vi "shell integration.vi"(7 "Command":enum16{"Add", "Remove"}(ring)=enum."Remove", 8 "error in":errorcluster, 11 "Cluster":T1={"App Key"="Test Key", "Context Label"="Test File Roottt", "Command"="Cmd", "Position"=enum."Middle", "Extended?"=FALSE, "Location"=enum."File - Root", "Icon path"="\"C:\\Users\\sajam\\LabVIEW Projects\\Personal projects\\Rename Extension\\Source Code\\rename.ico\"", "Ext (No Dot)"="Test"}) -> (0 "error out":errorcluster, 3 "Cluster":T1={"App Key"="Test Key", "Context Label"="Test Command", "Command"="none", "Position"=enum."Middle", "Extended?"=FALSE, "Location"=enum."Ext - Classes", "Icon path"="\"C:\\Users\\sajam\\LabVIEW Projects\\Personal projects\\Rename Extension\\Source Code\\rename.ico\"", "Ext (No Dot)"="Test"})   [LabVIEW 2023, in "User Interface.lvlib"]
uses:
  User Interface.lvlib
  Controls/registry settings cluster.ctl
  <vilib>/registry/registry.llb/Registry RtKey.ctl
  <vilib>/registry/registry.llb/Write Registry Value Simple STR.vi
panel:
  out "standard error":string
  out "standard output":string
  out "String":string
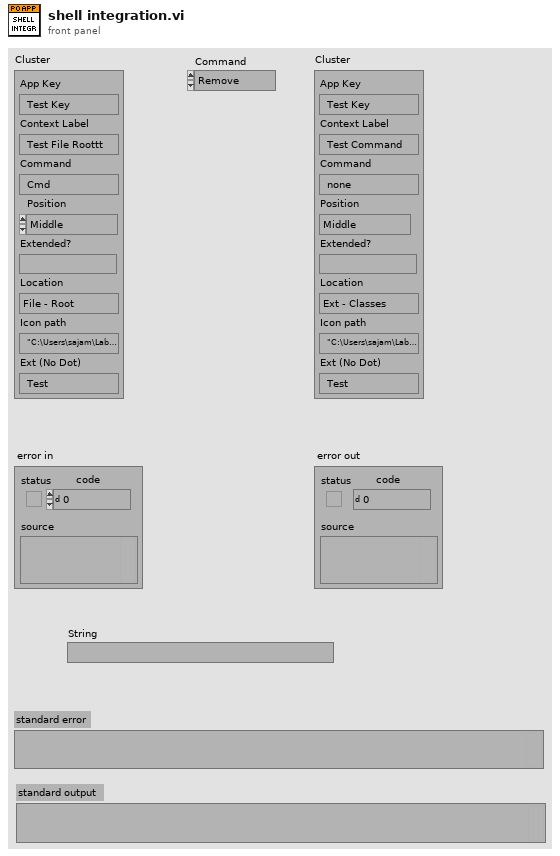
[diagram p1: front panel]
types:
  T1 = typedef "User Interface.lvlib/registry settings cluster.ctl" = cluster{"App Key":string, "Context Label":string, "Command":string, "Position":enum16{"Top", "Middle", "Bottom"}, "Extended?":bool, "Location":enum16{"File - Root", "Ext - Root", "Directory - Root", "File - Classes", "Ext - Classes", "Folder - Classes", "Dir Bak Gnd - Root"}, "Icon path":string, "Ext (No Dot)":string}
  T2 = typedef "Registry RtKey.ctl" = enum32{"HKEY_CLASSES_ROOT", "HKEY_CURRENT_USER", "HKEY_LOCAL_MACHINE", "HKEY_USERS", "HKEY_PERFORMANCE_DATA", "HKEY_CURRENT_CONFIG", "HKEY_DYN_DATA"}
  T3 = enum16{"File - Root", "Ext - Root", "Directory - Root", "File - Classes", "Ext - Classes", "Folder - Classes", "Dir Bak Gnd - Root"}
  T4 = typedef "Registry refnum.ctl" = refnum<k1>
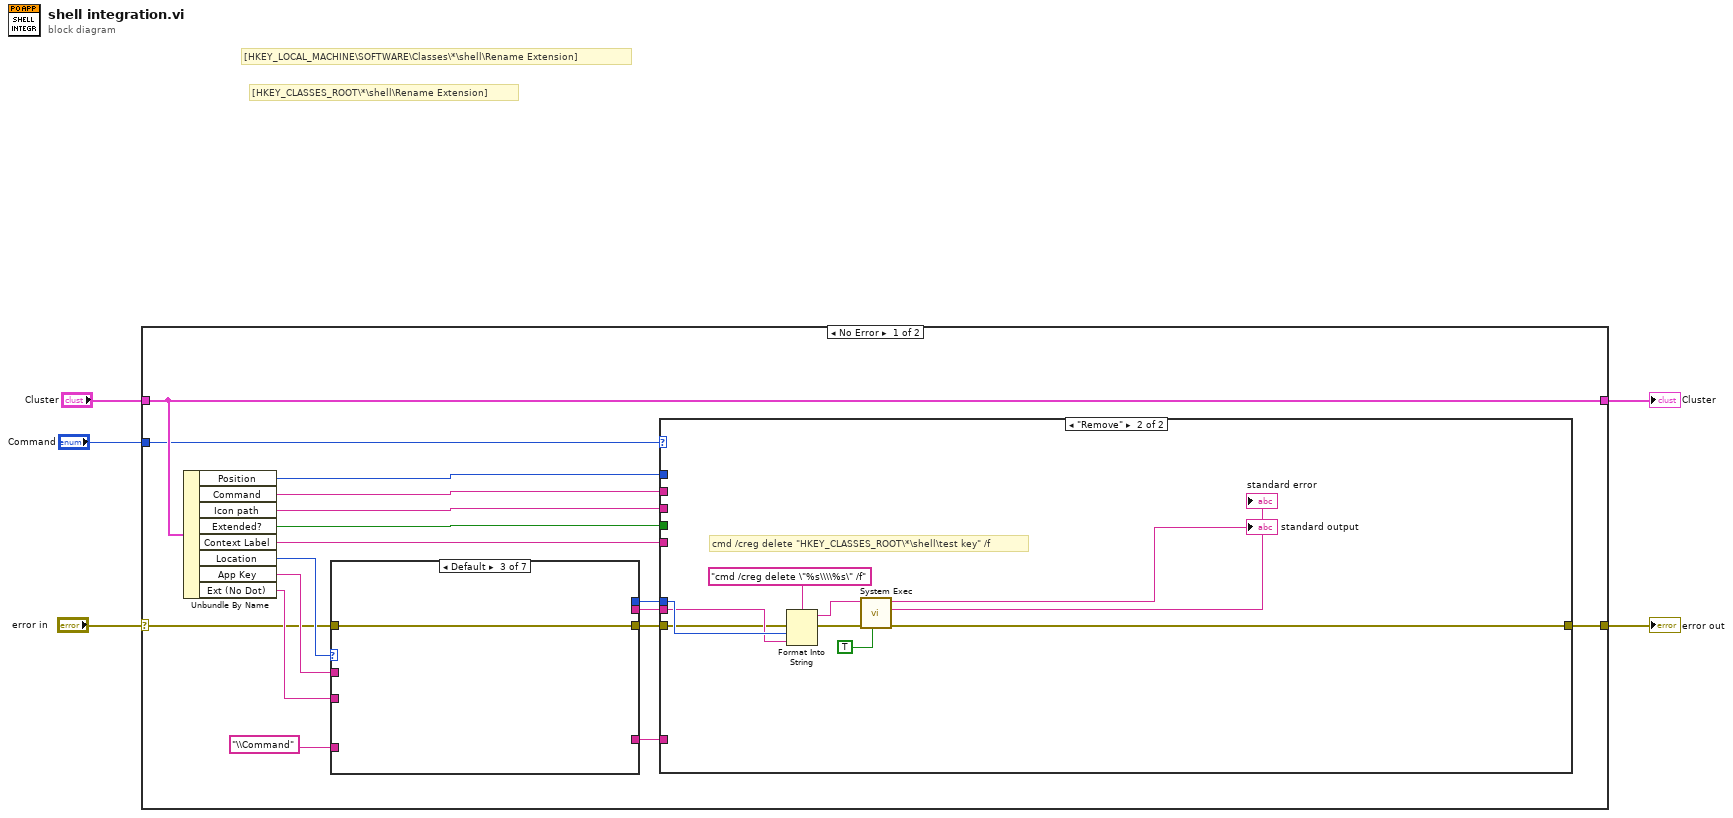
[diagram p0: block diagram]
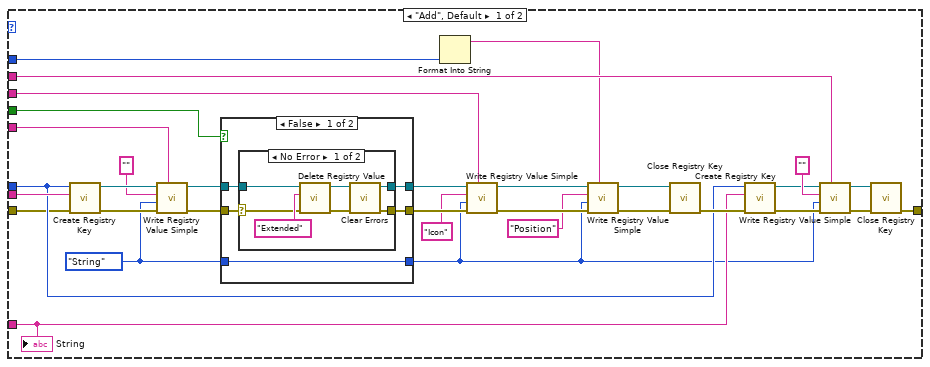
[diagram p2: hidden frame]
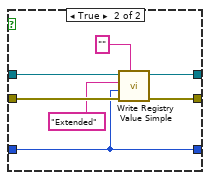
[diagram p4: hidden frame]
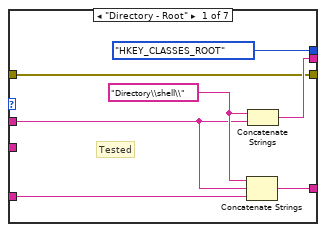
[diagram p5: hidden frame]
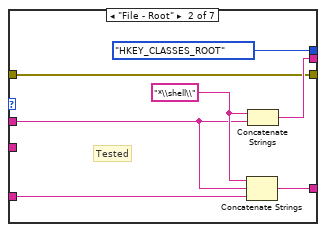
[diagram p6: hidden frame]
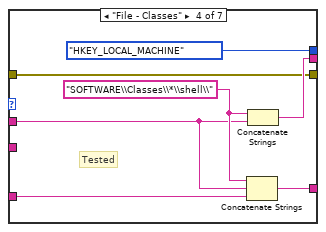
[diagram p7: hidden frame]
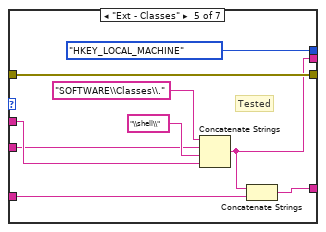
[diagram p8: hidden frame]
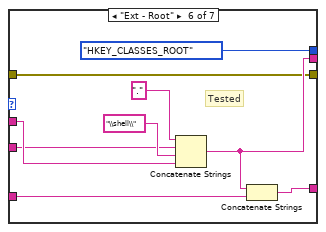
[diagram p9: hidden frame]
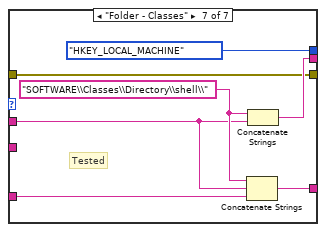
[diagram p10: hidden frame]
diagram:
  # "[HKEY_CLASSES_ROOT\\*\\shell\\Rename Extension]"
  # "[HKEY_LOCAL_MACHINE\\SOFTWARE\\Classes\\*\\shell\\Rename Extension]"
  n1 = case shown="No Error" "error in" {
    selector: "error in" -> [w9 w133]
    tunnel: "Cluster" -> [w8 w132]
    tunnel: [w6 w133] -> w4
    tunnel: [w8 w132] -> w2
    tunnel: "Command" -> [w7 _]
    frame No Error {
      n2 = Unbundle By Name(w8) -> ("Position"=w10:enum16{"Top", "Middle", "Bottom"}, "Command"=w15:string, "Icon path"=w14:string, "Extended?"=w18:bool, "Context Label"=w19:string, "Location"=w21:T3, "App Key"=w20:string, "Ext (No Dot)"=w12:string)
      n3 = case shown="Default" w21 {
        tunnel: [Registry_RtKey."HKEY_CLASSES_ROOT" ("root key (HKEY_LOCAL_MACHINE)") Registry_RtKey."HKEY_CLASSES_ROOT" ("root key (HKEY_LOCAL_MACHINE)") _ Registry_RtKey."HKEY_LOCAL_MACHINE" ("root key (HKEY_LOCAL_MACHINE)") Registry_RtKey."HKEY_LOCAL_MACHINE" ("root key (HKEY_LOCAL_MACHINE)") Registry_RtKey."HKEY_CLASSES_ROOT" ("root key (HKEY_LOCAL_MACHINE)") Registry_RtKey."HKEY_LOCAL_MACHINE" ("root key (HKEY_LOCAL_MACHINE)")] -> w17
        tunnel: [w90 w97 _ w105 w107 w117 w130] -> w22
        tunnel: w20 -> [w88 w95 _ w103 w113 w122 w128]
        tunnel: [w87 w94 _ w102 w112 w121 w127] -> w16
        tunnel: "\\Command" ("string") -> [w86 w93 _ w101 w111 w120 w126]
        tunnel: w12 -> [_ _ _ _ w110 w118 _]
        tunnel: w9 -> [w85 w92 w99 w100 w108 w116 w125]
        tunnel: [w85 w92 w99 w100 w108 w116 w125] -> w11
        frame "Directory - Root" {
          w89 = "Directory\\shell\\" ("subkey")
          # "Tested"
          n4 = Concatenate Strings(w89, w88, w86) -> (w87:string)
          n5 = Concatenate Strings(w89, w88) -> (w90:string)
        }
        frame "File - Root" {
          w96 = "*\\shell\\" ("subkey")
          # "Tested"
          n6 = Concatenate Strings(w96, w95, w93) -> (w94:string)
          n7 = Concatenate Strings(w96, w95) -> (w97:string)
        }
        frame Default {
        }
        frame "File - Classes" {
          w104 = "SOFTWARE\\Classes\\*\\shell\\" ("subkey")
          # "Tested"
          n8 = Concatenate Strings(w104, w103, w101) -> (w102:string)
          n9 = Concatenate Strings(w104, w103) -> (w105:string)
        }
        frame "Ext - Classes" {
          # "Tested"
          n10 = Concatenate Strings("SOFTWARE\\Classes\\." ("subkey"), w110, "\\shell\\" ("subkey"), w113) -> (w107:string)
          n11 = Concatenate Strings(w107, w111) -> (w112:string)
        }
        frame "Ext - Root" {
          # "Tested"
          n12 = Concatenate Strings("." ("subkey"), w118, "\\shell\\" ("subkey"), w122) -> (w117:string)
          n13 = Concatenate Strings(w117, w120) -> (w121:string)
        }
        frame "Folder - Classes" {
          w129 = "SOFTWARE\\Classes\\Directory\\shell\\" ("subkey")
          # "Tested"
          n14 = Concatenate Strings(w129, w128, w126) -> (w127:string)
          n15 = Concatenate Strings(w129, w128) -> (w130:string)
        }
      }
      n16 = case shown="\"Remove\"" w7 {
        tunnel: w22 -> [w54 w80]
        tunnel: w19 -> [w51 _]
        tunnel: w18 -> [w48 _]
        tunnel: w17 -> [w39 w81]
        tunnel: w16 -> [w38 _]
        tunnel: w15 -> [w36 _]
        tunnel: [w23 w77] -> w6
        tunnel: w14 -> [w35 _]
        tunnel: w11 -> [w34 w79]
        tunnel: w10 -> [w29 _]
        frame "Add", Default {
          w47 = enum16{"String", "Binary", "DWORD"}."String" ("simple data type")
          n17 = call <vilib>:"Create Registry Key.vi"("error in (no error)"=w34, "subkey"=w54, "root key (HKEY_LOCAL_MACHINE)"=w39) -> ("error out"=w52:errorcluster, "refnum out"=w53:T4)  [unwired: 6 in, 1 out]
          n18 = call-poly <vilib>:"Write Registry Value Simple.vi"("String/Binary data"=w51, "error in (no error)"=w52, "simple data type"=w47, "value"="", "refnum"=w53) -> ("error out"=w49:errorcluster, "refnum out"=w50:T4)  [unwired: 3 in]
          n19 = case shown="False" w48 {
            tunnel: w50 -> [w57 w74]
            tunnel: w49 -> [w58 w73]
            tunnel: [w56 w71] -> w45
            tunnel: [w55 w70] -> w46
            tunnel: w47 -> [w59 w69]
            tunnel: [w59 w69] -> w26
            frame False {
              n20 = case shown="No Error" w58 {
                selector: w58 -> [w60 w67]
                tunnel: w57 -> [w64 w66]
                tunnel: [w63 w66] -> w56
                tunnel: [w61 w67] -> w55
                frame No Error {
                  n21 = call <vilib>:"Delete Registry Value.vi"("error in (no error)"=w60, "value"="Extended", "refnum"=w64) -> ("error out"=w65:errorcluster, "refnum out"=w63:T4)  [unwired: 7 in]
                  n22 = call <vilib>:"Clear Errors.vi"("error in (no error)"=w65) -> ("error out"=w61:errorcluster)  [unwired: 5 in, 1 out]
                }
                frame Error {
                }
              }
            }
            frame True {
              n23 = call-poly <vilib>:"Write Registry Value Simple.vi"("String/Binary data"="", "error in (no error)"=w73, "simple data type"=w69, "value"="Extended", "refnum"=w74) -> ("error out"=w70:errorcluster, "refnum out"=w71:T4)  [unwired: 3 in]
            }
          }
          n24 = Format Into String(w29) -> (resulting string=w28:string)  [unwired: 3 in, 1 out]
          n25 = call-poly <vilib>:"Write Registry Value Simple.vi"("String/Binary data"=w35, "error in (no error)"=w46, "simple data type"=w26, "value"="Icon", "refnum"=w45) -> ("error out"=w33:errorcluster, "refnum out"=w31:T4)  [unwired: 3 in]
          n26 = call-poly <vilib>:"Write Registry Value Simple.vi"("String/Binary data"=w28, "error in (no error)"=w33, "simple data type"=w26, "value"="Position", "refnum"=w31) -> ("error out"=w32:errorcluster, "refnum out"=w30:T4)  [unwired: 3 in]
          n27 = call <vilib>:"Close Registry Key.vi"("error in (no error)"=w32, "refnum"=w30) -> ("error out"=w40:errorcluster)  [unwired: 5 in]
          n28 = call <vilib>:"Create Registry Key.vi"("error in (no error)"=w40, "subkey"=w38, "root key (HKEY_LOCAL_MACHINE)"=w39) -> ("error out"=w37:errorcluster, "refnum out"=w41:T4)  [unwired: 6 in, 1 out]
          n29 = call-poly <vilib>:"Write Registry Value Simple.vi"("String/Binary data"=w36, "error in (no error)"=w37, "simple data type"=w26, "value"="", "refnum"=w41) -> ("error out"=w24:errorcluster, "refnum out"=w25:T4)  [unwired: 3 in]
          n30 = call <vilib>:"Close Registry Key.vi"("error in (no error)"=w24, "refnum"=w25) -> ("error out"=w23:errorcluster)  [unwired: 5 in]
          "String" <- w38
        }
        frame "Remove" {
          # "cmd /creg delete \"HKEY_CLASSES_ROOT\\*\\shell\\test key\" /f"
          n31 = Format Into String(format string="cmd /creg delete \"%s\\\\%s\" /f", error in=w79, w81, w80) -> (resulting string=w76:string, error out=w78:errorcluster)  [unwired: 1 in]
          n32 = call <vilib>:"System Exec.vi"("run minimized? (F)"=TRUE, "error in (no error)"=w78, "command line"=w76) -> ("error out"=w77:errorcluster, "standard error"=→"standard error":string, "standard output"=→"standard output":string)  [unwired: 5 in, 1 out]
        }
      }
    }
    frame Error {
    }
  }
  "error out" <- w4
  "Cluster" <- w2
